vi "BonOMM-SAOMM.Test.vi"() -> ()   [LabVIEW 2011] (continued)
                                n4156 = local write "Offset Y"(w2454) -> ()
                                n4157 = local write "Offset Z"(w2453) -> ()
                                n4158 = local write "Offset U"(w2452) -> ()
                                n4159 = local write "Offset V"(w2451) -> ()
                                n4160 = case shown="True" w2406 {
                                tunnel: w2402 -> [_ w2464]
                                frame False {
                                }
                                frame True {
                                "Flux Max" <- w2464
                                }
                                }
                                n4161 = case shown="True" w2403 {
                                tunnel: w2402 -> [_ w2463]
                                frame False {
                                }
                                frame True {
                                "Flux Min" <- w2463
                                }
                                }
                                n4162 = To Double Precision Float(number=w2461) -> (double precision float=w2427:dbl)
                                n4163 = To Double Precision Float(number=w2459) -> (double precision float=w2429:dbl)
                                n4164 = Add(x=w2427, y=w2460) -> (x+y=w2411:dbl)
                                n4165 = Add(x=w2429, y=w2458) -> (x+y=w2410:dbl)
                                n4166 = local write "XCentroid"(w2411) -> ()
                                n4167 = Add(x=w2427, y=w2428) -> (x+y=w2412:dbl)
                                n4168 = Add(x=w2429, y=w2430) -> (x+y=w2409:dbl)
                                n4169 = Index Array(array=w2437) -> (element #1=→"Cmd X":dbl, element #2=→"Cmd Y":dbl, element #3=→"Cmd Z":dbl, element #4=→"Cmd U":dbl, element #5=→"Cmd V":dbl)  [unwired: 5 in]
                                n4170 = local write "YCentroid"(w2410) -> ()
                                n4171 = local write "XReference"(w2412) -> ()
                                n4172 = local write "YReference"(w2409) -> ()
                                n4173 = Subtract(x=w2412, y=w2411) -> (x-y=w2407:dbl)
                                n4174 = Subtract(x=w2409, y=w2410) -> (x-y=w2408:dbl)
                                n4175 = local write "DiffX"(w2407) -> ()
                                n4176 = local write "DiffY"(w2408) -> ()
                              }
                              frame #1 {
                                # "À terme, il faudra ici que l'écart soit :\n\n- Opération fixe : Hpos - Hoff\n- En boucle ouverte : Hpos - (Hlut + Hoff)\n- En asservissement : Hpos - (HOff)"
                                n4177 = local read "H_Offset"() -> (w2468:dbl[])
                                n4178 = local read "H_LUT"() -> (w2469:dbl[])
                                n4179 = local read "H_Position"() -> (w2470:dbl[])
                                n4180 = Add(x=w2469, y=w2468) -> (x+y=w2467:dbl[])
                                n4181 = Subtract(x=w2470, y=w2467) -> (x-y=w2471:dbl[])
                                n4182 = Index Array(array=w2471) -> (element #1=→"EcartX":dbl, element #2=→"EcartY":dbl, element #3=→"EcartZ":dbl, element #4=→"EcartU":dbl, element #5=→"EcartV":dbl)  [unwired: 5 in]
                              }
                              frame #2 {
                                # "ServoLevel = -1 si inactif ..."
                                # "Update des graphiques de guidage"
                                n4183 = Unbundle By Name(w2491) -> ("ServoLevel"=w2487:u16, "ROIXOffset"=w2497:u16, "CentroidX"=w2498:dbl, "Pixel X"=w2499:dbl, "ROIYOffset"=w2500:u16, "CentroidY"=w2501:dbl, "Pixel Y"=w2502:dbl)
                                n4184 = Unbundle By Name(w2491) -> ("SNR"=w2495:dbl, "SNRTreshold"=w2494:dbl, "Flux"=w2496:dbl)
                                n4185 = local read "Servo"() -> (w2486:bool)
                                n4186 = Boolean To (0,1)(Boolean=w2486) -> (0, 1=w2489:i16)
                                n4187 = Greater Than 0?(x=w2487) -> (x > 0?=w2488:bool)
                                n4188 = local read "CentroidsData"() -> (w2481:cluster{dbl[], dbl[]}[])
                                n4189 = local read "SNRData"() -> (w2480:cluster{dbl[], dbl[]}[])
                                n4190 = local read "FluxData"() -> (w2479:cluster{dbl[], dbl[]}[])
                                n4191 = Decrement(x=w2489) -> (x-1=w2485:i16)
                                n4192 = Bundle("SNR"=w2495, "SNRTreshold"=w2494, "Flux"=w2496) -> (w2492:T57)  [unwired: 1 in]
                                n4193 = To Unsigned Word Integer(number=w2485) -> (unsigned 16bit integer=w2484:u16)
                                n4194 = Select(t=w2487, s=w2488, f=w2484) -> (s? t:f=w2483:u16)
                                n4195 = Bundle("ServoLevel"=w2483, "ROIXOffset"=w2497, "CentroidX"=w2498, "Pixel X"=w2499, "ROIYOffset"=w2500, "CentroidY"=w2501, "Pixel Y"=w2502) -> (w2493:T58)  [unwired: 1 in]
                                n4196 = call "SAOMM-Graph-Guiding.vi"("SNR Data"=w2492, "TimeStamp"=w2475, "DataLenght (seconds)"=w2490, "Centroids Data"=w2493, "SNR IN"=w2480, "Flux IN"=w2479, "Centroids IN"=w2481) -> ("SNR OUT"=w2477:cluster{dbl[], dbl[]}[], "Flux OUT"=w2476:cluster{dbl[], dbl[]}[], "Centroids OUT"=w2478:cluster{dbl[], dbl[]}[])  [unwired: 6 in]
                                "SNRData" <- w2477
                                "FluxData" <- w2476
                                "CentroidsData" <- w2478
                                n4197 = local read "Servo"() -> (w2482:bool)
                                n4198 = case shown="True" w2482 {
                                tunnel: w2477 -> [_ w2539]
                                tunnel: w2476 -> [_ w2537]
                                tunnel: w2478 -> [_ w2542]
                                frame False {
                                }
                                frame True {
                                w2513 = 100.0 ("y")
                                n4199 = local read "GraphTimeStamp"() -> (w2535:dbl)
                                n4200 = Array Subset(array=w2542, index=0, length=2) -> (w2536:cluster{dbl[], dbl[]}[])
                                n4201 = local read "Binning"() -> (w2528:u16)
                                n4202 = local read "PixScale1"() -> (w2527:dbl)
                                n4203 = call "TroncateGraphData.vi"("TimeStampTreshold"=w2535, "Data IN"=w2539) -> ("Truncated Data"=→"Graph-SNR":cluster{dbl[], dbl[]}[])  [unwired: 13 in]
                                n4204 = call "TroncateGraphData.vi"("TimeStampTreshold"=w2535, "Data IN"=w2537) -> ("Truncated Data"=w2518:cluster{dbl[], dbl[]}[])  [unwired: 13 in]
                                n4205 = call "TroncateGraphData.vi"("TimeStampTreshold"=w2535, "Data IN"=w2536) -> ("Truncated Data"=w2534:cluster{dbl[], dbl[]}[])  [unwired: 13 in]
                                n4206 = To Double Precision Float(number=w2528) -> (double precision float=w2529:dbl)
                                n4207 = Index Array(array=w2534) -> (element #1=w2532:cluster{dbl[], dbl[]}, element #2=w2533:cluster{dbl[], dbl[]})  [unwired: 2 in]
                                n4208 = Index Array(array=w2518) -> (element #1=w2511:cluster{dbl[], dbl[]}, element #2=w2512:cluster{dbl[], dbl[]})  [unwired: 2 in]
                                n4209 = Multiply(x=w2529, y=w2527) -> (x*y=w2526:dbl)
                                n4210 = local read "Flux Max"() -> (w2508:dbl)
                                n4211 = Unbundle(w2532) -> (w2524:dbl[], w2531:dbl[])
                                n4212 = Unbundle(w2533) -> (w2525:dbl[], w2530:dbl[])
                                n4213 = Unbundle(w2511) -> (w2515:dbl[], w2510:dbl[])
                                n4214 = Unbundle(w2512) -> (w2514:dbl[], w2509:dbl[])
                                n4215 = Multiply(x=w2531, y=w2526) -> (x*y=w2523:dbl[])
                                n4216 = Multiply(x=w2530, y=w2526) -> (x*y=w2522:dbl[])
                                n4217 = Bundle(w2524, w2523) -> (w2520:cluster{dbl[], dbl[]})  [unwired: 1 in]
                                n4218 = Bundle(w2525, w2522) -> (w2521:cluster{dbl[], dbl[]})  [unwired: 1 in]
                                n4219 = Divide(x=w2510, y=w2508) -> (x/y=w2507:dbl[])
                                n4220 = Divide(x=w2509, y=w2508) -> (x/y=w2506:dbl[])
                                n4221 = Build Array(w2520, w2521) -> (→"Graph-Centroids":cluster{dbl[], dbl[]}[])
                                n4222 = Multiply(x=w2507, y=w2513) -> (x*y=w2516:dbl[])
                                n4223 = Multiply(x=w2506, y=w2513) -> (x*y=w2517:dbl[])
                                n4224 = Bundle(w2515, w2516) -> (w2505:cluster{dbl[], dbl[]})  [unwired: 1 in]
                                n4225 = Bundle(w2514, w2517) -> (w2504:cluster{dbl[], dbl[]})  [unwired: 1 in]
                                n4226 = Build Array(w2505, w2504) -> (→"Graph-Flux":cluster{dbl[], dbl[]}[])
                                }
                                }
                              }
                              frame #3 {
                                # "Update des graphiques de l'hexapode"
                                n4227 = local read "CumulativeError"() -> (w2543:cluster{dbl[], dbl[]}[])
                                n4228 = local read "HexXData"() -> (w2550:cluster{dbl[], dbl[]}[])
                                n4229 = local read "HexYData"() -> (w2549:cluster{dbl[], dbl[]}[])
                                n4230 = call "SAOMM-Graph-Hexapode.vi"("Hexapod cluster"=w2552, "LoggingTimeStamp"=w2545, "DataLenght (seconds)"=w2551, "X IN"=w2550, "Y IN"=w2549, "Cumul IN"=w2543) -> ("X OUT"=w2548:cluster{dbl[], dbl[]}[], "Y OUT"=w2547:cluster{dbl[], dbl[]}[], "Cumul OUT"=w2544:cluster{dbl[], dbl[]}[])  [unwired: 7 in]
                                "HexXData" <- w2548
                                "HexYData" <- w2547
                                "CumulativeError" <- w2544
                                n4231 = local read "Servo"() -> (w2546:bool)
                                n4232 = case shown="True" w2546 {
                                tunnel: w2548 -> [_ w2559]
                                tunnel: w2547 -> [_ w2558]
                                tunnel: w2544 -> [_ w2554]
                                frame False {
                                }
                                frame True {
                                n4233 = local read "GraphTimeStamp"() -> (w2553:dbl)
                                n4234 = call "TroncateGraphData.vi"("TimeStampTreshold"=w2553, "Data IN"=w2559) -> ("Truncated Data"=→"Hex-XGraph":cluster{dbl[], dbl[]}[])  [unwired: 13 in]
                                n4235 = call "TroncateGraphData.vi"("TimeStampTreshold"=w2553, "Data IN"=w2558) -> ("Truncated Data"=→"Hex-YGraph":cluster{dbl[], dbl[]}[])  [unwired: 13 in]
                                n4236 = call "TroncateGraphData.vi"("TimeStampTreshold"=w2553, "Data IN"=w2554) -> ("Truncated Data"=→"Cumulatif":cluster{dbl[], dbl[]}[])  [unwired: 13 in]
                                }
                                }
                              }
                            }
                          }
                        }
                      }
                    }
                  }
                }
              }
              frame #1 {
                n4237 = Wait (ms)(milliseconds to wait=u32 5) -> ()  [unwired: 1 out]
              }
            }
            n4238 = Tick Count (ms)() -> (millisecond timer value=w2068:u32)
            n4239 = Subtract(x=w2068, y=w2067) -> (x-y=→"ListenerExec":u32)
            n4240 = local read "Archivage SAOMM"() -> (w2058:bool)
            n4241 = local read "PrAMS + SAOMM"() -> (w2059:bool)
            n4242 = local read "Quit"() -> (w2060:bool)
            n4243 = Compound Arithmetic op=AND(w2058, w2059, w2060) -> (w2061:bool)
          }
          "PrAMS Listener" <- w948
          n4244 = while {
            shift-right: [w3425] -> _
            shift-left: w960 -> [w3424]
            shift-left: w960 -> [w3423]
            tunnel: [w3410] -> w953
            i -> [w3411]
            stop <- w3410 stop-if-true
            # "Optimisé pour f=5Hz"
            # "Structure de gestion des itérations périodiques"
            n4245 = local read "Hexapod COMM"() -> (w3412:bool)
            n4246 = Subtract(x=w3424, y=w3423) -> (x-y=→"TimeBetweenExec":u32)
            n4247 = local read "ExCmd COMM"() -> (w3416:bool)
            n4248 = local read "PrAMS COMM"() -> (w3415:bool)
            n4249 = local read "Calib COMM"() -> (w3417:bool)
            n4250 = local read "MCB COMM"() -> (w3413:bool)
            n4251 = local read "TCS COMM"() -> (w3414:bool)
            n4252 = local read "TableCOM"() -> (w3418:bool)
            n4253 = local read "MovingZ"() -> (w3419:bool)
            n4254 = local read "MovingXY"() -> (w3420:bool)
            n4255 = stacked-sequence {
              seq-local: [w3426 _ _ _ _ _ _ _ _ _ _ _] -> [_ _ _ _ _ _ _ _ _ _ _ w3869]
              seq-local: [_ w3455 _ _ _ _ _ _ _ _ _ _] -> [_ _ w3518 w3535 _ _ _ _ _ _ _ _]
              seq-local: [_ _ w3519 _ _ _ _ _ _ _ _ _] -> [_ _ _ _ w3605 _ _ _ _ _ _ _]
              seq-local: [_ _ _ w3536 _ _ _ _ _ _ _ _] -> [_ _ _ _ _ _ _ _ _ _ _ _]
              seq-local: [_ _ _ _ w3606 _ _ _ _ _ _ _] -> [_ _ _ _ _ _ w3665 _ _ _ _ _]
              seq-local: [_ _ _ _ _ _ w3664 _ _ _ _ _] -> [_ _ _ _ _ _ _ _ _ _ w3826 _]
              seq-local: [_ _ _ _ _ _ _ _ _ _ w3825 _] -> [_ _ _ _ _ _ _ _ _ _ _ _]
              seq-local: [_ _ _ _ _ _ _ _ w3673 _ _ _] -> [_ _ _ _ _ _ _ _ _ _ _ w3866]
              seq-local: [_ _ _ _ _ _ _ w3668 _ _ _ _] -> [_ _ _ _ _ _ _ _ w3672 _ _ _]
              seq-local: [_ _ _ _ _ _ _ w3667 _ _ _ _] -> [_ _ _ _ _ _ _ _ w3671 _ _ _]
              seq-local: [_ _ _ _ _ _ _ w3666 _ _ _ _] -> [_ _ _ _ _ _ _ _ w3670 _ _ _]
              tunnel: w3420 -> [_ _ _ _ _ _ _ _ _ w3712 _ _]
              tunnel: w3419 -> [_ _ _ _ _ _ _ _ _ w3708 _ _]
              tunnel: w3418 -> [_ w3454 _ _ _ _ _ _ _ _ _ _]
              tunnel: w3417 -> [_ w3453 _ _ _ _ _ _ _ _ _ _]
              tunnel: w3416 -> [_ w3452 _ _ _ _ _ _ _ _ _ _]
              tunnel: w3415 -> [_ w3451 _ _ _ _ _ _ _ _ _ _]
              tunnel: w3414 -> [_ w3450 _ _ _ _ _ _ _ _ _ _]
              tunnel: w3413 -> [_ w3449 _ _ _ _ _ _ _ _ _ _]
              tunnel: w3412 -> [_ w3439 _ _ _ _ _ _ _ _ _ _]
              tunnel: w3411 -> [_ w3431 _ _ _ _ _ _ _ _ _ _]
              frame #0 {
                n4256 = Tick Count (ms)() -> (millisecond timer value=w3426:u32)
              }
              frame #1 {
                w3438 = "-1" ("y")
                w3461 = "-1" ("y")
                w3464 = "-1" ("y")
                w3465 = "-1" ("y")
                w3468 = "-1" ("y")
                w3469 = "-1" ("y")
                w3473 = "-1" ("y")
                # "Update le menu s'il y a lieu ..."
                # "Vérification des erreurs de communications"
                n4257 = local read "MC-BonOMM VRN"() -> (w3456:refnum<visa-resource-name>)
                n4258 = local read "Hexapod VRN"() -> (w3436:refnum<visa-resource-name>)
                n4259 = local read "PrAMS VRN"() -> (w3458:refnum<visa-resource-name>)
                n4260 = local read "Excmd VRN"() -> (w3459:refnum<visa-resource-name>)
                n4261 = local read "Table VRN"() -> (w3471:refnum<visa-resource-name>)
                n4262 = local read "Calib VRN"() -> (w3460:refnum<visa-resource-name>)
                n4263 = local read "TCS VRN"() -> (w3457:refnum<visa-resource-name>)
                n4264 = Build Array(w3454, w3453, w3452, w3451, w3450, w3449, w3439) -> (w3443:bool[])
                n4265 = Boolean Array To Number(Boolean array=w3443) -> (number=w3440:u32)
                n4266 = Type Cast(type=w3438, x=w3436) -> (*(type *) &x=w3437:string)
                n4267 = Type Cast(type=w3473, x=w3471) -> (*(type *) &x=w3472:string)
                n4268 = Type Cast(type=w3469, x=w3460) -> (*(type *) &x=w3470:string)
                n4269 = Type Cast(type=w3468, x=w3459) -> (*(type *) &x=w3467:string)
                n4270 = Type Cast(type=w3465, x=w3458) -> (*(type *) &x=w3466:string)
                n4271 = Type Cast(type=w3464, x=w3457) -> (*(type *) &x=w3463:string)
                n4272 = Type Cast(type=w3461, x=w3456) -> (*(type *) &x=w3462:string)
                n4273 = Tick Count (ms)() -> (millisecond timer value=w3455:u32)
                n4274 = Not Equal?(x=w3437, y=w3438) -> (x != y?=w3435:bool)
                n4275 = Not Equal?(x=w3472, y=w3473) -> (x != y?=w3434:bool)
                n4276 = Not Equal?(x=w3470, y=w3469) -> (x != y?=w3448:bool)
                n4277 = Not Equal?(x=w3467, y=w3468) -> (x != y?=w3447:bool)
                n4278 = Not Equal?(x=w3466, y=w3465) -> (x != y?=w3446:bool)
                n4279 = Not Equal?(x=w3463, y=w3464) -> (x != y?=w3445:bool)
                n4280 = Not Equal?(x=w3462, y=w3461) -> (x != y?=w3444:bool)
                n4281 = case shown="False" w3434 {
                  frame False {
                    n4282 = local write "NeedOrigin"(TRUE ("Blinking")) -> ()
                  }
                  frame True {
                  }
                }
                n4283 = Build Array(w3434, w3448, w3447, w3446, w3445, w3444, w3435) -> (w3442:bool[])
                n4284 = Boolean Array To Number(Boolean array=w3442) -> (number=w3441:u32)
                n4285 = Not Equal?(x=w3441, y=w3440) -> (x != y?=w3433:bool)
                n4286 = Equal To 0?(x=w3431) -> (x = 0?=w3432:bool)
                n4287 = local read "ReconnectionMute"() -> (w3429:bool)
                n4288 = Or(x=w3433, y=w3432) -> (x .or. y?=w3430:bool)
                n4289 = Not(x=w3429) -> (.not. x?=w3428:bool)
                n4290 = And(x=w3428, y=w3430) -> (x .and. y?=w3427:bool)
                n4291 = case shown="True" w3427 {
                  tunnel: w3434 -> [_ w3513]
                  tunnel: w3448 -> [_ w3516]
                  tunnel: w3447 -> [_ w3515]
                  tunnel: w3446 -> [_ w3512]
                  tunnel: w3445 -> [_ w3510]
                  tunnel: w3444 -> [_ w3514]
                  tunnel: w3435 -> [_ w3511]
                  frame False {
                  }
                  frame True {
                    n4292 = Current VI's Menubar() -> (w3509:refnum<k9>)
                    n4293 = local write "TableCOM"(w3513) -> ()
                    n4294 = Set Menu Item Info(6:w3513, 7:"com_Tables de guidage" ("menu tag"), 11:w3509) -> (0:w3507:errorcluster, 3:w3508:refnum<k9>)  [unwired: 4 in]
                    n4295 = local write "Calib COMM"(w3516) -> ()
                    n4296 = Set Menu Item Info(6:w3516, 7:"com_Module de calibration" ("menu tag"), 8:w3507, 11:w3508) -> (0:w3505:errorcluster, 3:w3506:refnum<k9>)  [unwired: 3 in]
                    n4297 = local write "ExCmd COMM"(w3515) -> ()
                    n4298 = Set Menu Item Info(6:w3515, 7:"com_Commandes externes" ("menu tag"), 8:w3505, 11:w3506) -> (0:w3503:errorcluster, 3:w3504:refnum<k9>)  [unwired: 3 in]
                    n4299 = local write "PrAMS COMM"(w3512) -> ()
                    n4300 = Set Menu Item Info(6:w3512, 7:"com_Caméra de référence" ("menu tag"), 8:w3503, 11:w3504) -> (0:w3501:errorcluster, 3:w3502:refnum<k9>)  [unwired: 3 in]
                    n4301 = local write "TCS COMM"(w3510) -> ()
                    n4302 = Set Menu Item Info(6:w3510, 7:"com_Telescope Control System" ("menu tag"), 8:w3501, 11:w3502) -> (0:w3499:errorcluster, 3:w3500:refnum<k9>)  [unwired: 3 in]
                    n4303 = local write "MCB COMM"(w3514) -> ()
                    n4304 = Set Menu Item Info(6:w3514, 7:"com_MC-BonOMM" ("menu tag"), 8:w3499, 11:w3500) -> (0:w3478:errorcluster, 3:w3479:refnum<k9>)  [unwired: 3 in]
                    n4305 = local write "Hexapod COMM"(w3511) -> ()
                    n4306 = Set Menu Item Info(6:w3511, 7:"com_Secondaire Actif" ("menu tag"), 8:w3478, 11:w3479) -> (0:w3475:errorcluster, 3:w3476:refnum<k9>)  [unwired: 3 in]
                    n4307 = Set Menu Item Info(7:"main_Tables de guidage" ("menu tag"), 8:w3475, 9:w3513, 11:w3476) -> (0:w3484:errorcluster, 3:w3487:refnum<k9>)  [unwired: 3 in]
                    n4308 = Set Menu Item Info(7:"main_Secondaire Actif" ("menu tag"), 8:w3484, 9:w3511, 11:w3487) -> (0:w3480:errorcluster, 3:w3486:refnum<k9>)  [unwired: 3 in]
                    n4309 = Set Menu Item Info(7:"main_Caméra de référence" ("menu tag"), 8:w3480, 9:w3512, 11:w3486) -> (0:w3481:errorcluster, 3:w3482:refnum<k9>)  [unwired: 3 in]
                    n4310 = Set Menu Item Info(7:"main_Télescope" ("menu tag"), 8:w3481, 9:w3510, 11:w3482) -> (0:w3483:errorcluster, 3:w3485:refnum<k9>)  [unwired: 3 in]
                    n4311 = Set Menu Item Info(6:w3514, 7:"main_Roue à filtres" ("menu tag"), 8:w3483, 11:w3485) -> ()  [unwired: 3 in, 2 out]
                  }
                }
              }
              frame #2 {
                n4312 = Tick Count (ms)() -> (millisecond timer value=w3519:u32)
                n4313 = Subtract(x=w3519, y=w3518) -> (x-y=→"CommCheck":u32)
              }
              frame #3 {
                # "Update les registres d'état"
                n4314 = local read "TCS VRN"() -> (w3523:refnum<visa-resource-name>)
                n4315 = control-ref of="TCS actif"() -> (w3521:refnum<vi>)
                n4316 = local read "TCSMute"() -> (w3520:bool)
                n4317 = Tick Count (ms)() -> (millisecond timer value=w3536:u32)
                n4318 = case shown="False" w3520 {
                  tunnel: [w3552 w3554] -> w3543
                  tunnel: [w3551 w3554] -> w3542
                  tunnel: [w3550 w3554] -> w3541
                  tunnel: [w3549 w3554] -> w3540
                  tunnel: w3523 -> [w3547 w3553]
                  tunnel: [w3545 w3553] -> w3522
                  tunnel: w3521 -> [w3544 _]
                  frame False {
                    n4319 = call "EXCOM-26.vi"("VRN IN"=w3547, "Bool Refnum"=w3544) -> ("STATL"=w3552:bool[], "STATH"=w3551:bool[], "VRN OUT"=w3546:refnum<visa-resource-name>, "STATEX"=w3549:bool[], "STATLH"=w3550:bool[], "Error OUT"=w3548:errorcluster)  [unwired: 7 in, 1 out]
                    n4320 = call-poly "PolyCommError.vi"("VISA IN"=w3546, "error IN"=w3548) -> ("VISA OUT"=w3545:refnum<visa-resource-name>)  [unwired: 11 in, 2 out]
                  }
                  frame True {
                    w3554 = bool[] [] ("STATL")
                  }
                }
                n4321 = Subtract(x=w3536, y=w3535) -> (x-y=→"Wait4Flag":u32)
                n4322 = local write "Indicateur d'état"("Lecture du statut de TCS" ("Indicateur d'état")) -> ()
                n4323 = local read "Slewing"() -> (w3539:bool)
                n4324 = local read "Focus slew"() -> (w3538:bool)
                n4325 = local write "TCS VRN"(w3522) -> ()
                n4326 = flat-sequence {
                  tunnel: "Setting" -> [w3556]
                  tunnel: w3538 -> [w3557]
                  tunnel: w3539 -> [w3558]
                  tunnel: w3540 -> [w3559]
                  tunnel: w3541 -> [w3560]
                  tunnel: w3542 -> [w3561]
                  tunnel: w3543 -> [w3562]
                  tunnel: [w3562] -> w3532
                  tunnel: [w3561] -> w3531
                  tunnel: [w3560] -> w3530
                  tunnel: [w3559] -> w3529
                  tunnel: [w3558] -> w3528
                  tunnel: [w3557] -> w3527
                  tunnel: [w3556] -> w3526
                  tunnel: [w3555] -> w3525
                  tunnel: w3532 -> [w3596]
                  tunnel: w3531 -> [w3595]
                  tunnel: w3530 -> [w3594]
                  tunnel: w3529 -> [w3593]
                  tunnel: w3528 -> [w3592]
                  tunnel: w3527 -> [w3591]
                  tunnel: w3526 -> [w3590]
                  tunnel: w3525 -> [w3589]
                  tunnel: [w3589] -> w3524
                  tunnel: w3524 -> [w3602]
                  frame #0 {
                    n4327 = Tick Count (ms)() -> (millisecond timer value=w3555:u32)
                  }
                  frame #1 {
                    # "Détecte un déplacement du télescope"
                    # "Détecte un changement de focus"
                    # "Bits du statut du TCS"
                    n4328 = Index Array(array=w3593, index #1=2 ("Index"), index #2=0 ("Index")) -> (element #1=w3574:bool, element #2=w3577:bool)
                    "Mode Est" <- w3574
                    "Focus slew" <- w3577
                    n4329 = Index Array(array=w3595, index=4 ("Index")) -> (element=w3584:bool)
                    "Target OutofRange" <- w3584
                    n4330 = Index Array(array=w3595, index=0 ("Index")) -> (element=w3566:bool)
                    n4331 = Index Array(array=w3596, index=2 ("Index")) -> (element=→"Tracking":bool)
                    n4332 = Index Array(array=w3596, index=3 ("Index")) -> (element=→"Slew enabled":bool)
                    n4333 = Index Array(array=w3596, index=4 ("indice")) -> (element=w3582:bool)
                    n4334 = Index Array(array=w3596, index=5 ("Index")) -> (element=w3583:bool)
                    "Approaching limit" <- w3583
                    n4335 = Index Array(array=w3596, index=7 ("Index")) -> (element=w3568:bool)
                    "Slewing" <- w3568
                    n4336 = Not Equal?(x=w3566, y=w3590) -> (x != y?=w3567:bool)
                    n4337 = property on="Mode Inversé" class="Bool (strict)"("Visible"=w3574, "Blinking"=w3574) -> ()  [unwired: 2 in, 2 out]
                    n4338 = property on="Target OutofRange" class="Bool (strict)"("Visible"=w3584, "Blinking"=w3584) -> ()  [unwired: 2 in, 2 out]
                    n4339 = local write "Coupole-Tél"(w3582) -> ()
                    n4340 = Not Equal?(x=w3577, y=w3591) -> (x != y?=w3576:bool)
                    n4341 = property on="Approaching limit" class="Bool (strict)"("Visible"=w3583, "Blinking"=w3583) -> ()  [unwired: 2 in, 2 out]
                    n4342 = case shown="True" w3567 {
                      tunnel: w3566 -> [_ w3598]
                      frame False {
                      }
                      frame True {
                        n4343 = property on="Setting" class="Bool (strict)"("Val(Sgnl)"=w3598) -> ()  [unwired: 2 in, 2 out]
                      }
                    }
                    n4344 = case shown="True" w3576 {
                      tunnel: w3577 -> [_ w3599]
                      frame False {
                      }
                      frame True {
                        n4345 = property on="Focus slew" class="Bool (strict)"("Value (Signaling)"=w3599) -> ()  [unwired: 2 in, 2 out]
                      }
                    }
                    n4346 = Not Equal?(x=w3568, y=w3592) -> (x != y?=w3569:bool)
                    n4347 = property on="Slewing" class="Bool (strict)"("Blinking"=w3568) -> ()  [unwired: 2 in, 2 out]
                    n4348 = And(x=w3566, y=w3567) -> (x .and. y?=w3570:bool)
                    n4349 = And(x=w3568, y=w3569) -> (x .and. y?=w3571:bool)
                    n4350 = local read "Servo"() -> (w3563:bool)
                    n4351 = Or(x=w3570, y=w3571) -> (x .or. y?=w3564:bool)
                    n4352 = And(x=w3564, y=w3563) -> (x .and. y?=w3565:bool)
                    n4353 = case shown="True" w3565 {
                      selector: w3565 -> [_ w3597]
                      frame False {
                      }
                      frame True {
                        n4354 = property on="StopServo" class="Bool (strict)"("Val(Sgnl)"=w3597) -> ()  [unwired: 2 in, 2 out]
                      }
                    }
                    n4355 = case shown="True" w3569 {
                      tunnel: w3568 -> [_ w3600]
                      frame False {
                      }
                      frame True {
                        n4356 = property on="Slewing" class="Bool (strict)"("Value (Signaling)"=w3600) -> ()  [unwired: 2 in, 2 out]
                      }
                    }
                    "STATH" <- w3595
                    "STATLH" <- w3594
                    "STATEX" <- w3593
                    "STATL" <- w3596
                  }
                  frame #2 {
                    n4357 = Tick Count (ms)() -> (millisecond timer value=w3603:u32)
                    n4358 = Subtract(x=w3603, y=w3602) -> (x-y=→"TCS #26 (sort)":u32)
                  }
                }
              }
              frame #4 {
                n4359 = Tick Count (ms)() -> (millisecond timer value=w3606:u32)
                n4360 = Subtract(x=w3606, y=w3605) -> (x-y=→"TCS #26":u32)
              }
              frame #5 {
                # "Malheureusement, semble causé un problème \nquand on tente de reconnecté les tables ...\nChecher à comprendre c'Est avoir mal à la tête\nprobablement un VI non-réentrant partager entre\nle query de TCS et le query des tables ..."
                # "Patch pour l'angle (2013/06/22)\nÀ mettre au propre ... attention,\ncela à beaucoup d'impact sur beaucou\nde sous-routine ... (voir tout ce qui re-\nçoit l'angle à un moment)"
                # "À remettre dans un mode correct"
                n4361 = local read "TCSMute"() -> (w3607:bool)
                n4362 = local read "TCS VRN"() -> (w3620:refnum<visa-resource-name>)
                n4363 = control-ref of="TCS actif"() -> (w3618:refnum<vi>)
                n4364 = local read "dflt-EQX"() -> (w3617:dbl)
                n4365 = case shown="False" w3607 {
                  tunnel: [w3658 w3659] -> w3641
                  tunnel: [w3657 w3659] -> w3640
                  tunnel: [w3656 w3659] -> w3639
                  tunnel: [w3655 w3659] -> w3638
                  tunnel: [w3654 ""] -> w3637
                  tunnel: [w3653 w3659] -> w3630
                  tunnel: [w3652 w3659] -> w3629
                  tunnel: [w3651 w3659] -> w3628
                  tunnel: [w3650 w3659] -> w3627
                  tunnel: [w3649 errorcluster {"status"=FALSE, "code"=0, "source"=""} ("Error OUT")] -> w3626
                  tunnel: [w3648 w3662] -> w3621
                  tunnel: w3620 -> [w3647 w3662]
                  tunnel: w3618 -> [w3646 _]
                  tunnel: w3617 -> [w3645 _]
                  tunnel: [w3644 w3659] -> w3615
                  tunnel: [w3643 w3659] -> w3614
                  tunnel: [w3642 w3659] -> w3610
                  frame False {
                    n4366 = call "EXCOM-25-EQ.vi"("VISA resource name"=w3647, "Bool Refnum"=w3646, "Display Equinox"=w3645) -> ("HA"=w3655:dbl, "Q String"=w3654:string, "RA"=w3643:dbl, "Rotateur"=w3642:dbl, "DEC"=w3644:dbl, "Dome"=w3658:dbl, "Epoque"=w3653:dbl, "Focus"=w3657:dbl, "VISA resource name dup"=w3648:refnum<visa-resource-name>, "Masse d'air"=w3656:dbl, "Temps Sidéral"=w3652:dbl, "Temps Universel"=w3651:dbl, "Année"=w3650:dbl, "Error OUT"=w3649:errorcluster)  [unwired: 2 in, 1 out]
                  }
                  frame True {
                    w3659 = 0.0
                  }
                }
                "Q String" <- w3637
                "RA Tel" <- w3614
                "DEC Tel" <- w3615
                "Angle Hor." <- w3638
                "Epoch Tel" <- w3630
                "Air Mass" <- w3639
                "LST" <- w3629
                "UTC" <- w3628
                "AnnéeRL" <- w3627
                "Foyer" <- w3640
                "Coupole" <- w3641
                n4367 = call-poly "PolyCommError.vi"("VISA IN"=w3621, "error IN"=w3626) -> ("VISA OUT"=w3619:refnum<visa-resource-name>, "Error"=w3622:bool)  [unwired: 11 in, 1 out]
                n4368 = Not(x=w3622) -> (.not. x?=w3616:bool)
                n4369 = local write "Sync_Ready"(w3616) -> ()
                n4370 = Add(x=w3610, y="Ajustement fin de rotation") -> (x+y=w3609:dbl)
                "RotationTCS" <- w3609
                n4371 = local write "TCS VRN"(w3619) -> ()
                n4372 = Negate(x=w3609) -> (-x=w3613:dbl)
                n4373 = local read "N.O. Déc."() -> (w3632:string)
                n4374 = local read "N.O. A.D."() -> (w3634:string)
                n4375 = Add(x=w3613, y=90.0) -> (x+y=→"RotationEffective":dbl)
                n4376 = local read "NO epoch"() -> (w3631:dbl)
                n4377 = call "time-str-to-time-dbl-RA.vi"("Chaîne"=w3634) -> ("TCS_coords"=w3633:dbl)
                n4378 = call "time-str-to-time-dbl-DEC.vi"("Chaîne"=w3632) -> ("TCS_coords"=w3624:dbl)
                n4379 = expression code="x*3600"(w3633) -> (w3625:dbl)
                n4380 = expression code="x*3600"(w3624) -> (w3623:dbl)
                n4381 = call "Object_properties.vi"("Target RA"=w3625, "Target DEC"=w3623, "Target Epoch"=w3631, "Sideral Time"=w3629) -> ("NO HA"=w3636:dbl, "NO AM"=w3635:dbl)  [unwired: 7 in, 3 out]
                n4382 = local write "NO AM"(w3635) -> ()
                n4383 = local write "NO HA"(w3636) -> ()
              }
              frame #6 {
                n4384 = Tick Count (ms)() -> (millisecond timer value=w3664:u32)
                n4385 = Subtract(x=w3664, y=w3665) -> (x-y=→"TCS #25":u32)
              }
              frame #7 {
                n4386 = local read "Position X"() -> (w3668:dbl)
                n4387 = local read "Position Z"() -> (w3666:dbl)
                n4388 = local read "Position Y"() -> (w3667:dbl)
              }
              frame #8 {
                n4389 = Tick Count (ms)() -> (millisecond timer value=w3673:u32)
                n4390 = local read "TableMute"() -> (w3669:bool)
                n4391 = case shown="False" w3669 {
                  tunnel: w3672 -> [w3681 _]
                  tunnel: w3671 -> [w3680 _]
                  tunnel: w3670 -> [w3679 _]
                  frame False {
                    # "Si on tente une reconnexion, on empêche le query ..."
                    n4392 = local read "Table Error"() -> (w3689:errorcluster)
                    n4393 = local read "Table VRN"() -> (w3690:refnum<visa-resource-name>)
                    n4394 = control-ref of="Table actif"() -> (w3691:refnum<vi>)
                    n4395 = call "Newmark-QueryPosition.vi"("Table VRN IN"=w3690, "Bool Refnum"=w3691, "Error IN"=w3689) -> ("X Axis"=w3685:dbl, "Y Axis"=w3684:dbl, "Table VRN OUT"=w3688:refnum<visa-resource-name>, "Exception"=w3686:string, "Z Axis"=w3678:dbl, "Error OUT"=w3687:errorcluster)  [unwired: 5 in, 2 out]
                    "Position X" <- w3685
                    "Position Y" <- w3684
                    "Position Z" <- w3678
                    n4396 = flat-sequence {
                      tunnel: w3686 -> [w3698]
                      tunnel: [w3698] -> w3694
                      tunnel: w3694 -> [w3701]
                      frame #0 {
                        n4397 = control-ref of="Table actif"() -> (w3700:refnum<vi>)
                        n4398 = call "Newmark-Wait4Flag.vi"("Raise Flag ?"=TRUE, "Ctl Refnum IN"=w3700) -> ()  [unwired: 8 in, 2 out]
                      }
                      frame #1 {
                        n4399 = local read "Exceptions"() -> (w3703:T3)
                        n4400 = call "ExceptionStacker.vi"("ExceptionString"=w3701, "Newmark-Exceptions IN"=w3703) -> ("Newmark-Exceptions OUT"=w3702:T3)  [unwired: 13 in]
                        n4401 = local write "Exceptions"(w3702) -> ()
                      }
                      frame #2 {
                        n4402 = local write "Table actif"(FALSE ("Table actif")) -> ()
                      }
                    }
                    n4403 = Not Equal?(x=w3681, y=w3685) -> (x != y?=w3683:bool)
                    n4404 = Not Equal?(x=w3680, y=w3684) -> (x != y?=w3682:bool)
                    n4405 = local write "Table Error"(w3687) -> ()
                    n4406 = Or(x=w3683, y=w3682) -> (x .or. y?=w3674:bool)
                    n4407 = local write "Table VRN"(w3688) -> ()
                    n4408 = local write "MovingXY"(w3674) -> ()
                    n4409 = local write "Indicateur d'état"("Lecture des paramètres des tables" ("Indicateur d'état")) -> ()
                    n4410 = local write "FoyerTable"(w3678) -> ()
                    n4411 = Not Equal?(x=w3678, y=w3679) -> (x != y?=w3677:bool)
                    n4412 = local write "MovingZ"(w3677) -> ()
                    n4413 = local read "Origine en cours..."() -> (w3675:bool)
                    n4414 = Or(x=w3674, y=w3675) -> (x .or. y?=w3676:bool)
                    n4415 = case shown="True" w3676 {
                      frame False {
                        # "Désactive les boutons quand la position \ncible est différente de la position lue."
                        n4416 = local read "CorrectXY"() -> (w3695:bool)
                        n4417 = case shown="False" w3695 {
                          frame False {
                            w3696 = T17."Enabled" ("Disabled")
                            n4418 = property on="Centre" class="Bool (strict)"("Disabled"=w3696) -> ()  [unwired: 2 in, 2 out]
                            n4419 = property on="Alacible" class="Bool (strict)"("Disabled"=w3696) -> ()  [unwired: 2 in, 2 out]
                            n4420 = property on="Origine" class="Bool (strict)"("Disabled"=w3696) -> ()  [unwired: 2 in, 2 out]
                            n4421 = property on="go Est" class="Bool (strict)"("Disabled"=w3696) -> ()  [unwired: 2 in, 2 out]
                            n4422 = property on="Calibration" class="Bool (strict)"("Disabled"=w3696) -> ()  [unwired: 2 in, 2 out]
                            n4423 = property on="Centrage" class="Bool"("Disabled"=w3696) -> ()  [unwired: 2 in, 2 out]
                            n4424 = property on="go Sud" class="Bool (strict)"("Disabled"=w3696) -> ()  [unwired: 2 in, 2 out]
                            n4425 = property on="RangeTable" class="Bool (strict)"("Disabled"=w3696) -> ()  [unwired: 2 in, 2 out]
                            n4426 = property on="Foyer+" class="Bool (strict)"("DisabledEnum"=w3696) -> ()  [unwired: 2 in, 2 out]
                            n4427 = property on="go Ouest" class="Bool (strict)"("Disabled"=w3696) -> ()  [unwired: 2 in, 2 out]
                            n4428 = property on="Foyer-" class="Bool (strict)"("DisabledEnum"=w3696) -> ()  [unwired: 2 in, 2 out]
                            n4429 = property on="go Nord" class="Bool (strict)"("Disabled"=w3696) -> ()  [unwired: 2 in, 2 out]
                          }
                          frame True {
                          }
                        }
                      }
                      frame True {
                        w3697 = T17."Disabled and Grayed Out" ("Disabled")
                        n4430 = property on="Centre" class="Bool (strict)"("Disabled"=w3697) -> ()  [unwired: 2 in, 2 out]
                        n4431 = property on="Alacible" class="Bool (strict)"("Disabled"=w3697) -> ()  [unwired: 2 in, 2 out]
                        n4432 = property on="Origine" class="Bool (strict)"("Disabled"=w3697) -> ()  [unwired: 2 in, 2 out]
                        n4433 = property on="go Est" class="Bool (strict)"("Disabled"=w3697) -> ()  [unwired: 2 in, 2 out]
                        n4434 = property on="Calibration" class="Bool (strict)"("Disabled"=w3697) -> ()  [unwired: 2 in, 2 out]
                        n4435 = property on="Centrage" class="Bool"("Disabled"=w3697) -> ()  [unwired: 2 in, 2 out]
                        n4436 = property on="go Sud" class="Bool (strict)"("Disabled"=w3697) -> ()  [unwired: 2 in, 2 out]
                        n4437 = property on="RangeTable" class="Bool (strict)"("Disabled"=w3697) -> ()  [unwired: 2 in, 2 out]
                        n4438 = property on="Foyer+" class="Bool (strict)"("DisabledEnum"=w3697) -> ()  [unwired: 2 in, 2 out]
                        n4439 = property on="go Ouest" class="Bool (strict)"("Disabled"=w3697) -> ()  [unwired: 2 in, 2 out]
                        n4440 = property on="Foyer-" class="Bool (strict)"("DisabledEnum"=w3697) -> ()  [unwired: 2 in, 2 out]
                        n4441 = property on="go Nord" class="Bool (strict)"("Disabled"=w3697) -> ()  [unwired: 2 in, 2 out]
                      }
                    }
                    "TabQstr" <- ""
                  }
                  frame True {
                  }
                }
              }
              frame #9 {
                # "Détecte un arrêt du stage Z"
                # "Détecte un arrêt des tables XY\nMovingXY -> était vrai, devient faux"
                # "Détection de l'arrêt des tables de translation ..."
                n4442 = local read "MovingZ"() -> (w3706:bool)
                n4443 = local read "MovingXY"() -> (w3711:bool)
                n4444 = Not(x=w3706) -> (.not. x?=w3707:bool)
                n4445 = And(x=w3708, y=w3707) -> (x .and. y?=w3705:bool)
                n4446 = Not(x=w3711) -> (.not. x?=w3710:bool)
                n4447 = And(x=w3712, y=w3710) -> (x .and. y?=w3709:bool)
                n4448 = case shown="True" w3709 {
                  frame False {
                  }
                  frame True {
                    # "Détecte un arrêt des étages XY"
                    n4449 = flat-sequence {
                      frame #0 {
                        n4450 = local read "CorrectXY"() -> (w3733:bool)
                        n4451 = case shown="True" w3733 {
                          frame False {
                          }
                          frame True {
                            n4452 = local write "CorrectXY"(FALSE ("CorrectXY")) -> ()
                            n4453 = property on="ApplyCorrection" class="Bool (strict)"("Val(Sgnl)"=TRUE ("Value (Signaling)")) -> ()  [unwired: 2 in, 2 out]
                          }
                        }
                      }
                      frame #1 {
                        n4454 = local read "CurvCorrect"() -> (w3736:bool)
                        n4455 = case shown="True" w3736 {
                          frame False {
                          }
                          frame True {
                            n4456 = local read "CentreTel X"() -> (w3746:dbl)
                            n4457 = local read "CentreTel Y"() -> (w3745:dbl)
                            n4458 = local read "Position X"() -> (w3739:dbl)
                            n4459 = local read "Position Y"() -> (w3738:dbl)
                            n4460 = local read "FoyerAuCentre"() -> (w3742:dbl)
                            n4461 = call "Calc_focus.vi"("Pos X"=w3739, "a0"=w3742, "Pos Y"=w3738, "Cen X"=w3746, "Cen Y"=w3745, "a1"="a1_focus", "a2"="a2_focus", "a3"="a3_focus") -> ("Foyer"=w3744:dbl)  [unwired: 6 in, 1 out]
                            n4462 = local write "CurvCorrect"(FALSE ("CorrectZ")) -> ()
                            n4463 = property on="FoyerTable" class="DigNum (strict)"("Val(Sgnl)"=w3744) -> ()  [unwired: 2 in, 2 out]
                          }
                        }
                      }
                    }
                  }
                }
                n4464 = case shown="True" w3705 {
                  frame False {
                  }
                  frame True {
                    # "Détecte un arrêt de l'étage de foyer"
                    n4465 = flat-sequence {
                      tunnel: [w3714] -> w3713
                      tunnel: w3713 -> [w3721]
                      frame #0 {
                        n4466 = local read "CorrectZ"() -> (w3715:bool)
                        n4467 = case shown="True" w3715 {
                          tunnel: [w3716 w3717] -> w3714
                          frame False {
                            n4468 = local read "Position Z"() -> (w3716:dbl)
                          }
                          frame True {
                            n4469 = local read "Cible Z"() -> (w3717:dbl)
                            n4470 = local write "CorrectZ"(FALSE ("CorrectZ")) -> ()
                            n4471 = property on="ApplyCorrection" class="Bool (strict)"("Val(Sgnl)"=TRUE ("Value (Signaling)")) -> ()  [unwired: 2 in, 2 out]
                          }
                        }
                      }
                      frame #1 {
                        # "Ajuste le foyer en fonction du nombre de pas à partir du centre"
                        n4472 = local read "Focusing"() -> (w3720:bool)
                        n4473 = case shown="True" w3720 {
                          tunnel: w3721 -> [_ w3723]
                          frame False {
                          }
                          frame True {
                            n4474 = local read "Reference X"() -> (w3729:dbl)
                            n4475 = local read "Reference Y"() -> (w3730:dbl)
                            n4476 = local read "Position X"() -> (w3724:dbl)
                            n4477 = local read "Position Y"() -> (w3725:dbl)
                            n4478 = local read "a1_focus"() -> (w3731:dbl)
                            n4479 = local read "a2_focus"() -> (w3727:dbl)
                            n4480 = local read "a3_focus"() -> (w3728:dbl)
                            n4481 = call "Calc_focus.vi"("Pos X"=w3724, "Pos Y"=w3725, "Cen X"=w3729, "Cen Y"=w3730, "a1"=w3731, "a2"=w3727, "a3"=w3728) -> ("Residu"=w3726:dbl)  [unwired: 7 in, 1 out]
                            n4482 = Subtract(x=w3723, y=w3726) -> (x-y=w3732:dbl)
                            n4483 = local write "Focusing"(FALSE ("Focusing")) -> ()
                            n4484 = local write "FoyerAuCentre"(w3732) -> ()
                          }
                        }
                      }
                    }
                  }
                }
              }
              frame #10 {
                w3813 = u16 0 items=["Square", "Circle"] ("Ring")
                # "Calcul des astrométries et positions ..."
                # "Invert X"
                # "Redessine la représentation du champ"
                # "Réinitialise le data USNO"
                # "Réinitialise l'image"
                # "Vérifie si les données sont encore actuelles ..."
                # "Nombre d'arcsec\nd'écart acceptées"
                # "Époque DSS et USNO"
                # "Calcul la position de la sonde ..."
                # "Refait avec les nouvelles astrométries ..."
                n4485 = Tick Count (ms)() -> (millisecond timer value=w3825:u32)
                n4486 = Subtract(x=w3825, y=w3826) -> (x-y=→"Table Q":u32)
                n4487 = local read "Binning"() -> (w3761:u16)
                n4488 = local read "Dec Sonde"() -> (w3757:dbl)
                n4489 = local read "PixScale1"() -> (w3763:dbl)
                n4490 = local read "PixScale2"() -> (w3762:dbl)
                n4491 = local read "RA Sonde"() -> (w3758:dbl)
                n4492 = local read "Naxis1"() -> (w3764:u16)
                n4493 = local read "Naxis2"() -> (w3765:u16)
                n4494 = local read "RotationEffective"() -> (w3755:dbl)
                n4495 = local read "Reference Y"() -> (w3771:dbl)
                n4496 = local read "Reference X"() -> (w3772:dbl)
                n4497 = local read "RotationEffective"() -> (w3754:dbl)
                n4498 = local read "CentreTel X"() -> (w3774:dbl)
                n4499 = local read "CentreTel Y"() -> (w3773:dbl)
                n4500 = Bundle("Naxis1"=w3764, "Naxis2"=w3765) -> (w3759:cluster{"Naxis1":u16, "Naxis2":u16})  [unwired: 1 in]
                n4501 = Bundle("PixScale1"=w3763, "PixScale2"=w3762) -> (w3760:cluster{"PixScale1":dbl, "PixScale2":dbl})  [unwired: 1 in]
                n4502 = local read "arcsec/pulse"() -> (w3815:dbl)
                n4503 = call "SAOMM-Astrometry.vi"("Binning"=w3761, "PIXSCALE"=w3760, "NAXIS"=w3759, "Rotation"=w3755, "RAsonde"=w3758, "DECsonde"=w3757) -> ("GuideAstrom"=w3756:T4)  [unwired: 9 in]
                n4504 = local read "DEC Tel"() -> (w3818:dbl)
                n4505 = local read "RA Tel"() -> (w3819:dbl)
                n4506 = local write "GuiderAstrom"(w3756) -> ()
                n4507 = local read "Représentation"() -> (w3787:dbl)
                n4508 = property on="TableXYPos" class="XYGraph (strict)"("Active Cursor"=u32 1) -> ("Cursor.Cursor X"=w3749:dbl, "Cursor.Cursor Y"=w3748:dbl)  [unwired: 2 in, 2 out]
                n4509 = local read "MirVig"() -> (w3751:dbl)
                n4510 = local read "Miroir"() -> (w3750:dbl)
                n4511 = call "Set_field_astrometry.vi"("Cen x (pas)"=w3774, "effective rotation (°)"=w3754, "scale (\"/pas)"=w3815, "NaxisMax"=500000, "Cen y (pas)"=w3773, "Use Center?"=FALSE ("Ues Constant Size ?"), "Ref x (pas)"=w3772, "Ref y (pas)"=w3771, "RA (HH:MM:SS.S)"=w3819, "DEC(DD:MM:SS)"=w3818, "Inversion Cluster"=T20 {"Invert Angle"=FALSE, "Invert X"=TRUE, "Invert Y"=FALSE}) -> ("Field Astrometry"=w3811:T4, "Table Astrometry"=w3812:T4)  [unwired: 3 in]
                n4512 = local read "FOV"() -> (w3814:dbl)
                n4513 = Bundle("Miroir"=w3750, "Cursor.Cursor X"=w3749, "Cursor.Cursor Y"=w3748, "MirVig"=w3751) -> (w3747:T47)  [unwired: 1 in]
                n4514 = local read "NaxisMax"() -> (w3770:dbl)
                n4515 = call "draw_field.vi"("Field_Astrometry"=w3811, "FOV"=w3814, "NaxisMax"=w3770, "Ring"=w3813, "Table_Astrometry"=w3812, "Ues Constant Size ?"=TRUE, "margin/size"=w3787, "MirrorAvatar"=w3747) -> ("TableXYPos"=w3797:cluster{dbl[], dbl[]}[], "X Scale.Range"=w3798:T26, "ImgDEC"=w3753:dbl, "ImgRA"=w3808:dbl, "Y Scale.Range"=w3796:T26)  [unwired: 3 in]
                n4516 = local read "Epoch Tel"() -> (w3809:dbl)
                n4517 = local read "DEC-USNO"() -> (w3781:dbl)
                n4518 = local write "FieldAstrom"(w3811) -> ()
                n4519 = local write "TableAstrom"(w3812) -> ()
                n4520 = local read "RA-USNO"() -> (w3782:dbl)
                n4521 = local read "Position X"() -> (w3768:dbl)
                n4522 = local read "Position Y"() -> (w3767:dbl)
                n4523 = call "precess.vi"("Eq2"=2000.0, "Eq1"=w3809, "DEC 1"=w3753, "RA 1"=w3808) -> ("DEC 2"=w3785:dbl, "RA 2"=w3786:dbl)
                "RA-Champ" <- w3786
                "DEC-Champ" <- w3785
                n4524 = call "xy2ad.vi"("Y (px)"=w3767, "X (px)"=w3768, "Astrometry"=w3812) -> ("DEC (°)"=w3820:dbl, "RA (°)"=w3821:dbl, "DEC (HH:MM:SS)"=→"Dec Sonde":dbl, "RA (HH:MM:SS.S)"=→"RA Sonde":dbl)  [unwired: 5 in]
                n4525 = local read "Img DEC"() -> (w3775:dbl)
                n4526 = local read "Img RA"() -> (w3776:dbl)
                n4527 = call "deg2ad.vi"("DEC (°)"=w3785, "RA (°)"=w3786) -> ("DEC (°)"=→"DEC-Champ-sec":dbl, "RA (sec)"=→"RA-Champ-sec":dbl)
                n4528 = call "deg2ad.vi"("DEC (°)"=w3781, "RA (°)"=w3782) -> ("DEC (°)"=→"DEC-USNO-sec":dbl, "RA (sec)"=→"RA-USNO-sec":dbl)
                n4529 = flat-sequence {
                  tunnel: w3821 -> [w3851]
                  tunnel: w3820 -> [w3850]
                  tunnel: w3811 -> [w3849]
                  tunnel: [w3848] -> w3799
                  tunnel: w3798 -> [w3846]
                  tunnel: w3797 -> [w3845]
                  tunnel: w3796 -> [w3844]
                  tunnel: w3799 -> [w3853]
                  frame #0 {
                    # "Calcul la position de la cible"
                    n4530 = call "ad2xy.vi"("DEC"=w3850, "RA"=w3851, "Astrometry"=w3849) -> ("Y"=w3842:dbl, "X"=w3843:dbl, "Dup Astrometry"=w3848:T4)  [unwired: 6 in]
                    n4531 = call "format_arcmin2arcsecstr.vi"("RA arcmin"=w3843, "DEC Arcmin"=w3842) -> ("Formatted RA"=→"Cen-Snd-RA":string, "Formatted Dist"=→"Cen-Snd-TOT":string, "Formatted DEC"=→"Cen-Snd-DEC":string)  [unwired: 11 in]
                    n4532 = property on="TableXYPos" class="XYGraph (strict)"("Active Cursor"=u32 1, "Cursor.Cursor X"=w3843, "Cursor.Cursor Y"=w3842, "Value"=w3845, "XScale.Range"=w3846, "YScale.Range"=w3844) -> ()  [unwired: 2 in, 2 out]
                  }
                  frame #1 {
                    n4533 = case shown="False" "CursorLock" {
                      tunnel: w3853 -> [w3859 _]
                      frame False {
                        n4534 = property on="TableXYPos" class="XYGraph (strict)"("Active Cursor"=u32 0) -> ("Cursor.Cursor X"=w3858:dbl, "Cursor.Cursor Y"=w3857:dbl)  [unwired: 2 in, 2 out]
                        n4535 = call "format_arcmin2arcsecstr.vi"("RA arcmin"=w3858, "DEC Arcmin"=w3857) -> ("Formatted RA"=w3854:string, "Formatted Dist"=→"Cen-Cib-TOT":string, "Formatted DEC"=w3855:string)  [unwired: 11 in]
                        n4536 = call "xy2ad.vi"("Y (px)"=w3857, "X (px)"=w3858, "Astrometry"=w3859) -> ("DEC (HH:MM:SS)"=→"Dec Cible":dbl, "RA (HH:MM:SS.S)"=→"RA Cible":dbl)  [unwired: 5 in, 2 out]
                        n4537 = local write "Cen-Cib-RA"(w3854) -> ()
                        n4538 = local write "Cen-Cib-DEC"(w3855) -> ()
                      }
                      frame True {
                      }
                    }
                  }
                }
                n4539 = expression code="x/3600"(5.0) -> (w3789:dbl)
                n4540 = call "deg2ad.vi"("DEC (°)"=w3775, "RA (°)"=w3776) -> ("DEC (°)"=→"DEC-DSS-sec":dbl, "RA (sec)"=→"RA-DSS-sec":dbl)
                n4541 = Subtract(x=w3786, y=w3776) -> (x-y=w3807:dbl)
                n4542 = Subtract(x=w3786, y=w3782) -> (x-y=w3790:dbl)
                n4543 = Subtract(x=w3785, y=w3775) -> (x-y=w3806:dbl)
                n4544 = Subtract(x=w3785, y=w3781) -> (x-y=w3791:dbl)
                n4545 = Absolute Value(x=w3806) -> (abs(x)=w3803:dbl)
                n4546 = Absolute Value(x=w3791) -> (abs(x)=w3793:dbl)
                n4547 = Absolute Value(x=w3807) -> (abs(x)=w3805:dbl)
                n4548 = Absolute Value(x=w3790) -> (abs(x)=w3792:dbl)
                n4549 = Greater?(x=w3805, y=w3789) -> (0:w3802:bool)
                n4550 = Greater?(x=w3803, y=w3789) -> (0:w3801:bool)
                n4551 = Greater?(x=w3792, y=w3789) -> (0:w3794:bool)
                n4552 = Greater?(x=w3793, y=w3789) -> (0:w3795:bool)
                n4553 = Or(x=w3802, y=w3801) -> (x .or. y?=w3800:bool)
                n4554 = Or(x=w3794, y=w3795) -> (x .or. y?=w3788:bool)
                n4555 = case shown="True" w3788 {
                  frame False {
                  }
                  frame True {
                    w3832 = 0
                    n4556 = local read "SubIMG4DSS?"() -> (w3828:bool)
                    n4557 = local read "Integrating"() -> (w3830:bool)
                    n4558 = Initialize Array(sgl 0.0, w3832, w3832) -> (w3831:sgl[][])
                    n4559 = local write "BestTargetLed"(FALSE) -> ()
                    n4560 = local write "ImgData"(w3831) -> ()
                    n4561 = Not(x=w3830) -> (.not. x?=w3829:bool)
                    n4562 = And(x=w3828, y=w3829) -> (x .and. y?=w3827:bool)
                    n4563 = case shown="True" w3827 {
                      tunnel: w3831 -> [_ w3838]
                      frame False {
                      }
                      frame True {
                        w3835 = u16 2 items=["Region d'intérêt", "Prévisualisation", "Idle"] ("ImageUsage")
                        n4564 = call "Draw_crosshair.vi"("Image IN"=w3838, "White Value"=sgl 255.0) -> ("Image OUT"=w3837:sgl[][])  [unwired: 13 in]
                        n4565 = local write "ImageUsage"(w3835) -> ()
                        n4566 = local write "subimg"(w3837) -> ()
                      }
                    }
                  }
                }
                n4567 = case shown="True" w3800 {
                  frame False {
                  }
                  frame True {
                    w3863 = FALSE ("ImageDSSLed")
                    n4568 = local write "ImageDSSLed"(w3863) -> ()
                    n4569 = property on="TableXYPos" class="XYGraph (strict)"("PlotImages.Back"=picture data[5B] ("Plot Images:Back")) -> ()  [unwired: 2 in, 2 out]
                    n4570 = local write "DS9-Led"(w3863) -> ()
                  }
                }
              }
              frame #11 {
                # "Ajout des données des LVDTs"
                n4571 = Tick Count (ms)() -> (millisecond timer value=w3867:u32)
                n4572 = Subtract(x=w3867, y=w3869) -> (x-y=→"TotalExecTime":u32)
                n4573 = Subtract(x=w3867, y=w3866) -> (x-y=→"CursorSet":u32)
              }
            }
            n4574 = Wait Until Next ms Multiple(millisecond multiple=u32 200) -> ()  [unwired: 1 out]
            n4575 = local read "Quit"() -> (w3410:bool)
            n4576 = Tick Count (ms)() -> (millisecond timer value=w3425:u32)
          }
          "Query et Status" <- w953
          n4577 = while {
            tunnel: [w3167] -> w952
            i -> [w3168]
            stop <- w3167 stop-if-true
            # "À passer dans une boucle périodique à plusieurs étages parce que c'est le bordel."
            # "Structure de gestion des événements software"
            n4578 = event shown="[3] \"Slewing\": Value Change" {
              selector: _ -> [_ _ _ _]
              dyn-events: _ -> [_ _ _ _]
              timeout: 250 -> [_ _ _ _]
              tunnel: w3168 -> [w3171 _ _ _]
              event Timeout {
                # "Au ~30 sec ..."
                # "Reconnection/Acquisition des donneés météo ..."
                # "Au ~10 secondes ..."
                n4579 = event-data() -> ()  [unwired: 1 in, 2 out]
                n4580 = Quotient & Remainder(x=w3171, y=40) -> (x-y*floor(x/y)=w3175:i32)  [unwired: 1 out]
                n4581 = Equal To 0?(x=w3175) -> (x = 0?=w3174:bool)
                n4582 = case shown="True" w3174 {
                  frame False {
                  }
                  frame True {
                    n4583 = stacked-sequence {
                      frame #0 {
                        # "Si le foyer reste constant pendant plus de 5 minutes, on suppose que le foyer a été fait et est correct ..."
                        n4584 = local read "CheckFocus"() -> (w3183:bool)
                        n4585 = case shown="True" w3183 {
                          frame False {
                          }
                          frame True {
                            n4586 = local read "last_foc_chg"() -> (w3187:ext)
                            n4587 = Get Date/Time In Seconds() -> (seconds since 1Jan1904=w3189:timestamp)
                            n4588 = To Extended Precision Float(1:w3189) -> (0:w3188:ext)
                            n4589 = Subtract(x=w3188, y=w3187) -> (x-y=w3186:ext)
                            n4590 = Greater?(x=w3186, y=ext 300.0) -> (0:w3184:bool)
                            n4591 = case shown="True" w3184 {
                              frame False {
                              }
                              frame True {
                                # "Si il y a une connexion à\nla station météo ..."
                                # "Une fois que le comportement aura été testé, on pourra\nécrire le résultat dans le fichier \"instruments.ini\""
                                n4592 = local read "Cx"() -> (w3191:bool)
                                n4593 = case shown="True" w3191 {
                                frame False {
                                }
                                frame True {
                                # "On enregistre les données ..."
                                n4594 = local read "indic-T-out"() -> (w3193:dbl)
                                n4595 = local read "indic-T-in"() -> (w3192:dbl)
                                n4596 = local read "path_focuslog"() -> (w3194:path)
                                n4597 = local read "Instrument Actuel"() -> (w3195:string)
                                n4598 = local read "tmp.str"() -> (w3196:dbl)
                                n4599 = local read "Foyer Nominal"() -> (w3197:dbl)
                                n4600 = call "write_focus_file.vi"("Log_dir"=w3194, "Instrument"=w3195, "Foyer"=w3197, "Temp.str"=w3196, "Temp.int"=w3192, "Temp.ext"=w3193) -> ()  [unwired: 6 in]
                                n4601 = local read "Ath_coef"() -> (w3201:dbl)
                                n4602 = Multiply(x=w3201, y=w3196) -> (x*y=w3200:dbl)
                                n4603 = Subtract(x=w3197, y=w3200) -> (x-y=w3199:dbl)
                                n4604 = To Long Integer(number=w3199) -> (32bit integer=w3198:i32)
                                n4605 = local write "Foyer à 0°"(w3198) -> ()
                                }
                                }
                                n4606 = local write "CheckFocus"(FALSE ("CheckFocus")) -> ()
                              }
                            }
                          }
                        }
                      }
                      frame #1 {
                        # "Modification du foyer par une \ndifférence de température ..."
                        # "Éventuellement à calculer à partir\ndes données instrumentales ..."
                        n4607 = local read "indic-T-struct"() -> (w3207:dbl)
                        n4608 = local read "tmp.str"() -> (w3202:dbl)
                        n4609 = local read "Bypass Auto-focus"() -> (w3208:bool)
